vi "WRITE LINE CSV.vi"(10 "Array":string[](array[string]), 11 "FIle Ref":refnum<file>) -> (3 "Byte Stream File out":refnum<file>)   [LabVIEW 2016]
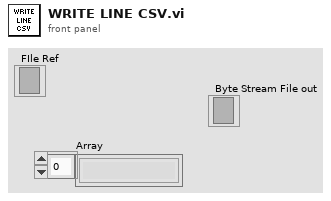
[diagram p1: front panel]
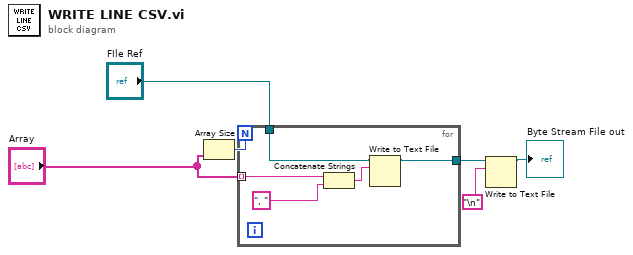
[diagram p0: block diagram]
diagram:
  n1 = Array Size(array="Array") -> (size(s)=w2:i32)
  n2 = for {
    N: w2 -> [_]
    tunnel: "FIle Ref" -> [w9]
    tunnel: "Array" -> [w11] mode=indexing
    tunnel: [w8] -> w4
    n3 = Concatenate Strings(w11, ", ") -> (w10:string)
    n4 = Write to Text File(file (use dialog)=w9, text=w10) -> (refnum out=w8:refnum<file>)  [unwired: 2 in, 2 out]
  }
  n5 = Write to Text File(file (use dialog)=w4, text="\n") -> (refnum out=→"Byte Stream File out":refnum<file>)  [unwired: 2 in, 2 out]
